vi "UIRef.vi"(8 "error in":errorcluster, 11 "node in":refnum<class "VIPB Build Node.lvclass">) -> (0 "error out":errorcluster, 2 "VI refnum":refnum<vi>, 3 "node out":refnum<class "VIPB Build Node.lvclass">)   [LabVIEW 2014, in "VIPB Build Node.lvclass"]
doc: "Stores the static reference to the UI of the node.Copyright 2015 National Instruments Corporation\n\nLicensed under the Apache License, Version 2.0 (the \"License\"); you may not use this file except in compliance with the License. You may obtain a copy of the License at http://www.apache.org/licenses/LICENSE-2.0\nUnless required by applicable law or agreed to in writing, software distributed under the License is distributed on an \"AS IS\" BASIS, WITHOUT WARRANTIES OR CONDITIONS OF ANY KIND, either express or implied. See the License for the specific language governing permissions and limitations under the License."
uses:
  VIPB Build Node.lvclass
  VIPB Build UI.vi
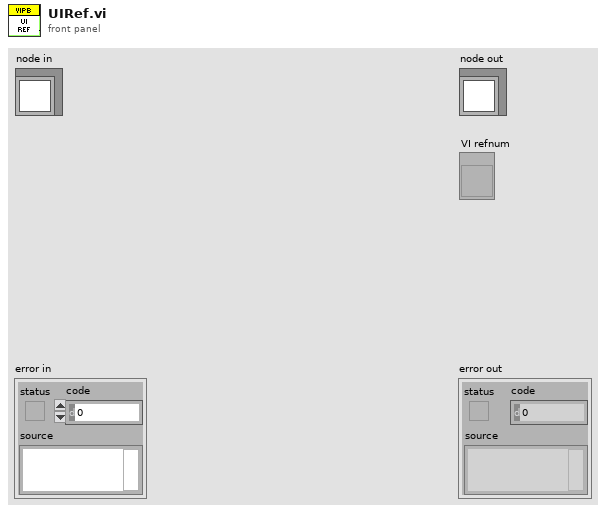
[diagram p1: front panel]
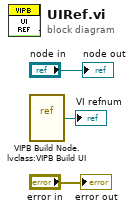
[diagram p0: block diagram]
diagram:
  n1 = vi-ref "VIPB Build Node.lvclass:VIPB Build UI.vi"() -> (→"VI refnum":refnum<vi>)
  "error out" <- "error in"
  "node out" <- "node in"
